vi "Process design.vi"(8 "error in (no error)":errorcluster, 9 "progress":refnum<vi>, 10 "Request Pending":bool, 11 "DesignRequest":T1) -> (0 "design error":errorcluster, 1 "output error":errorcluster, 2 "DesignRequest out":T1, 3 "Mathcad Output":T2, 5 "Find-Replace":cluster{"Find":string, "Replace":string}[](array[cluster]))   [LabVIEW 2012, in "Design Server.lvlib"]
uses:
  Design Server.lvlib
  Design Request.ctl
  Variable cluster.ctl
  AutoCAD cmds.ctl
  Word cmd.ctl
  Mathcad15 cmds.ctl
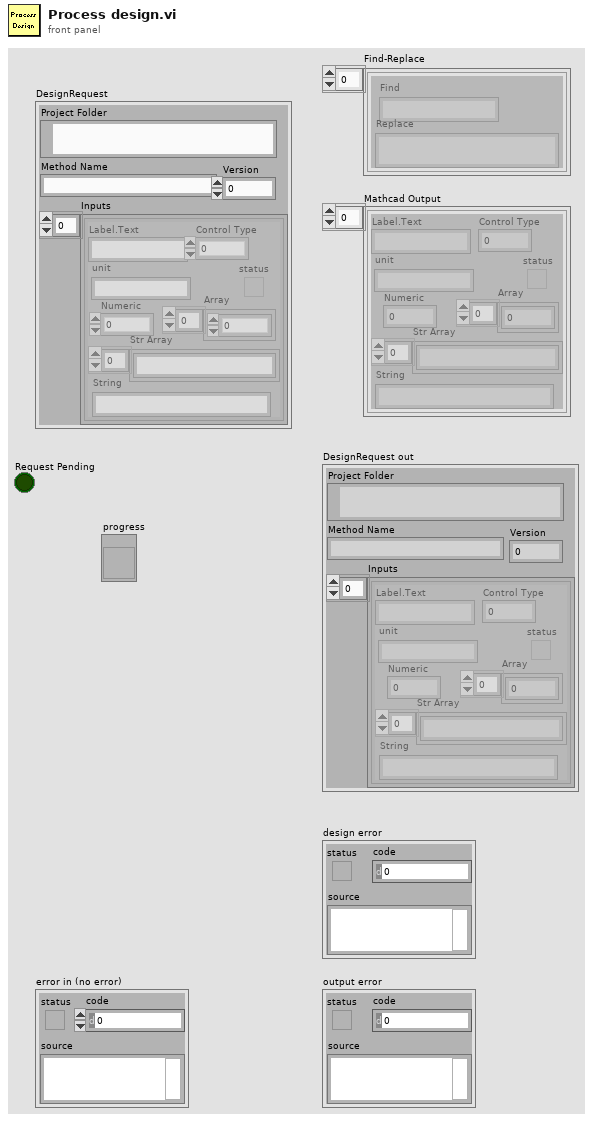
[diagram p1: front panel]
types:
  T1 = typedef "Design Server.lvlib/Design Request.ctl" = cluster{"Project Folder":path, "Method Name":string, "Inputs":T2, "Version":i32}
  T2 = typedef "Design Server.lvlib/Variable cluster.ctl" = cluster{"Label.Text":string, "Control Type":u32, "Numeric":dbl, "Array":dbl[], "status":bool, "Str Array":string[], "String":string, "unit":string}[]
  T3 = typedef "Design Server.lvlib/Mathcad15 cmds.ctl" = enum16{"Open Mathcad", "Execute Method", "Quit Mathcad"}
  T4 = typedef "Design Server.lvlib/Word cmd.ctl" = enum16{"Initialize", "Create Reports", "Quit"}
  T5 = typedef "Design Server.lvlib/AutoCAD cmds.ctl" = enum16{"Open AutoCAD", "Create Drawing", "Quit"}
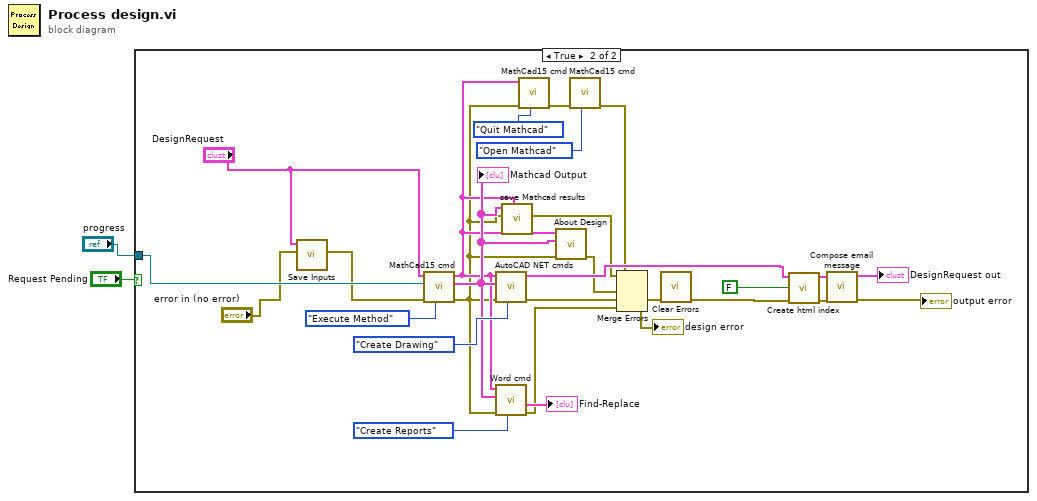
[diagram p0: block diagram]
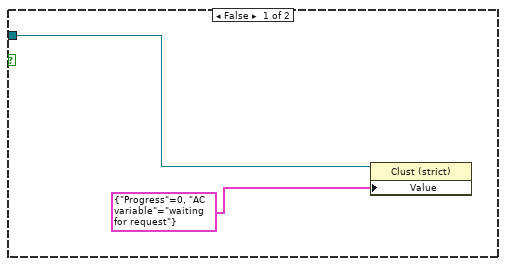
[diagram p2: hidden frame]
diagram:
  n1 = case shown="True" "Request Pending" {
    tunnel: "progress" -> [w3 w29]
    frame False {
      n2 = property class="Clust (strict)"(reference=w3, "Value"=cluster{"Progress":u8, "AC variable":string} {"Progress"=0, "AC variable"="waiting for request"} ("progress")) -> ()  [unwired: 1 in, 2 out]
    }
    frame True {
      n3 = call "Save Inputs.vi"("error in"="error in (no error)", "DesignRequest"="DesignRequest") -> ("error out"=w10:errorcluster)  [unwired: 9 in]
      n4 = call "MathCad15 cmd.vi"("Mathcad15 cmds"=Mathcad15_cmds."Execute Method", "error in"=w10, "progress"=w29, "DesignRequest"="DesignRequest") -> ("first error out"=w6:errorcluster, "Mathcad Output"=w8:T2, "DesignRequest out"=w7:T1)  [unwired: 5 in]
      "Mathcad Output" <- w8
      n5 = call "AutoCAD NET cmds.vi"("AutoCAD cmd"=AutoCAD_cmds."Create Drawing", "error in (no error)"=w6, "Mathcad Output"=w8, "DesignRequest"=w7) -> ("error out"=w16:errorcluster, "DesignRequest out"=w26:T1)  [unwired: 6 in]
      n6 = call "Word cmd.vi"("Word cmd"=Word_cmd."Create Reports", "Error In (no error)"=w6, "Mathcad Output"=w8, "DesignRequest"=w7) -> ("error out"=w18:errorcluster, "Find-Replace"=→"Find-Replace":cluster{"Find":string, "Replace":string}[])  [unwired: 6 in]
      n7 = call "save Mathcad results.vi"("DesignRequest"=w7, "error in"=w6, "MathCAD results"=w8) -> ("error out"=w5:errorcluster)  [unwired: 8 in]
      n8 = call "MathCad15 cmd.vi"("Mathcad15 cmds"=Mathcad15_cmds."Quit Mathcad", "error in"=w6, "DesignRequest"=w7) -> ("first error out"=w22:errorcluster)  [unwired: 6 in, 2 out]
      n9 = call "About Design.vi"("error in"=w6, "Mathcad Output"=w8, "DesignRequest"=w7) -> ("error out"=w9:errorcluster)  [unwired: 8 in]
      n10 = call "MathCad15 cmd.vi"("Mathcad15 cmds"=Mathcad15_cmds."Open Mathcad", "error in"=w22) -> ("first error out"=w13:errorcluster)  [unwired: 7 in, 2 out]
      n11 = Merge Errors(w5, w13, w9, w16, w18) -> (w23:errorcluster)
      "design error" <- w23
      n12 = call <vilib>:"Clear Errors.vi"("error in (no error)"=w23) -> ("error out"=w25:errorcluster)  [unwired: 6 in]
      n13 = call "Create html index.vi"("error in"=w25, "Under construction"=FALSE, "DesignRequest"=w26) -> ("error out"=w28:errorcluster, "DesignRequest out"=w27:T1)  [unwired: 7 in]
      n14 = call "Compose email message.vi"("error in (no error)"=w28, "DesignRequest"=w27) -> ("error out"=→"output error":errorcluster, "DesignRequest out"=→"DesignRequest out":T1)  [unwired: 8 in]
    }
  }
